vi "Write Parallel Operation Period(ms).vi"(8 "error in (no error)":errorcluster, 10 "Parallel Operation Period(ms)":i32=100, 11 "Parallel Operation Actor in":refnum<class "Parallel Operation Actor.lvclass">) -> (0 "error out":errorcluster, 3 "Parallel Operation Actor out":refnum<class "Parallel Operation Actor.lvclass">)   [LabVIEW 2024, in "Parallel Operation Actor.lvclass"]
uses:
  Parallel Operation Actor.lvclass
  Parallel Operation Actor.lvclass/Parallel Operation Actor.ctl
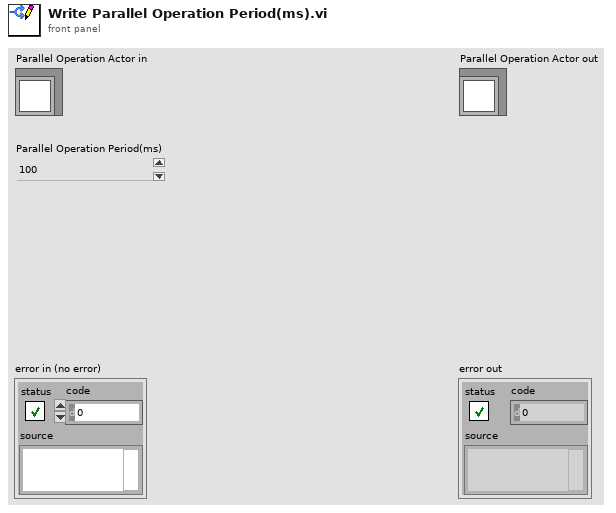
[diagram p1: front panel]
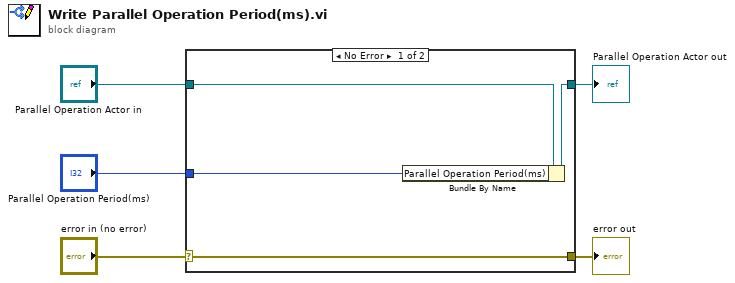
[diagram p0: block diagram]
diagram:
  n1 = case shown="No Error" "error in (no error)" {
    selector: "error in (no error)" -> [w9 w10]
    tunnel: [w9 w10] -> w4
    tunnel: [w7 w11] -> w2
    tunnel: "Parallel Operation Actor in" -> [w8 w11]
    tunnel: "Parallel Operation Period(ms)" -> [w6 _]
    frame No Error {
      n2 = Bundle By Name(cluster=w8, "Parallel Operation Period(ms)"=w6) -> (w7:refnum<class "Parallel Operation Actor.lvclass">)
    }
    frame Error {
    }
  }
  "error out" <- w4
  "Parallel Operation Actor out" <- w2
